vi "Close Tags.vi"(8 "error in (no error)":errorcluster, 11 "Logger in.lvclass":refnum<class "Logger.lvclass">) -> (0 "error out":errorcluster, 3 "Logger out.lvclass":refnum<class "Logger.lvclass">)   [LabVIEW 2017, in "Logger.lvclass"]
uses:
  Logger.lvclass
  Logger.lvclass/Logger.ctl
  <vilib>/Skyline/Tag/Wrapper/Wrapper_class/NI Skyline Tag.lvclass
  <vilib>/Skyline/Tag/Wrapper/Wrapper_class/Close Tag (Multiple).vi
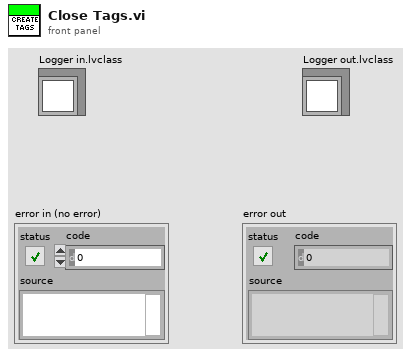
[diagram p1: front panel]
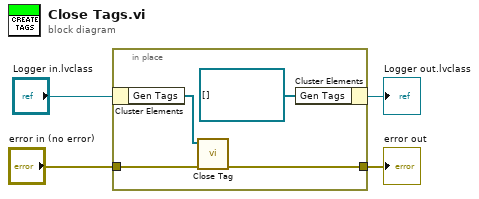
[diagram p0: block diagram]
diagram:
  n1 = in-place {
    in-place-border: "error in (no error)" -> [w6]
    in-place-border: [w5] -> w1
    n2 = in-place-cluster #1("Logger in.lvclass") -> ("Gen Tags"=w8:refnum<class "NI Skyline Tag.lvclass">[])
    n3 = call-poly <vilib>:"Close Tag.vi"("error in (no error)"=w6, "tags in"=w8) -> ("error out"=w5:errorcluster)  [unwired: 9 in]
    n4 = in-place-cluster #1("Gen Tags"=refnum<class "NI Skyline Tag.lvclass">[] []) -> (→"Logger out.lvclass":refnum<class "Logger.lvclass">)
  }
  "error out" <- w1
